vi "Close Group.vi"(8 "error in":errorcluster, 10 "Group":string, 11 "TDMS in":refnum<class "TDMS.lvclass">) -> (0 "error out":errorcluster, 3 "TDMS out":refnum<class "TDMS.lvclass">)   [LabVIEW 2019, in "TDMS.lvlib" / "TDMS.lvclass"]
uses:
  TDMS.lvclass
  TDMS.lvclass/TDMS.ctl
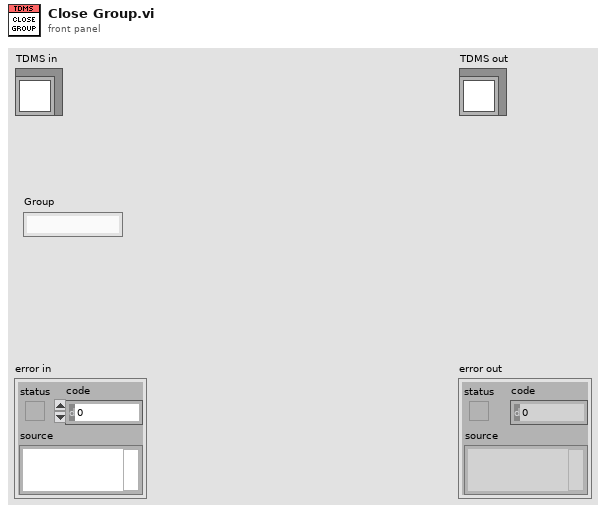
[diagram p1: front panel]
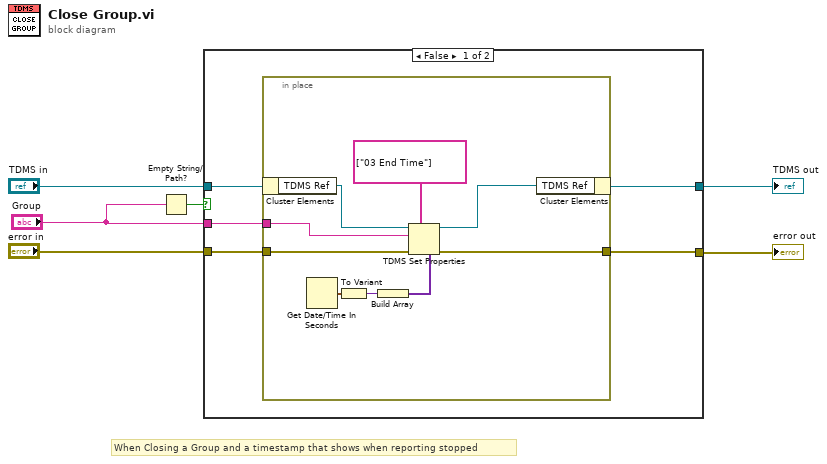
[diagram p0: block diagram]
diagram:
  # "When Closing a Group and a timestamp that shows when reporting stopped"
  n1 = Empty String/Path?(string/path="Group") -> (empty?=w2:bool)
  n2 = case shown="False" w2 {
    tunnel: [w11 w22] -> w6
    tunnel: "error in" -> [w10 w21]
    tunnel: [w9 w21] -> w4
    tunnel: "TDMS in" -> [w8 w22]
    tunnel: "Group" -> [w7 _]
    frame False {
      n3 = in-place {
        in-place-border: w10 -> [w16]
        in-place-border: [w18] -> w9
        in-place-border: w7 -> [w12]
        n4 = in-place-cluster #1(w8) -> ("TDMS Ref"=w20:refnum<k34>)
        n5 = Get Date/Time In Seconds() -> (seconds since 1Jan1904=w15:timestamp)
        n6 = To Variant(anything=w15) -> (Variant=w14:variant)
        n7 = Build Array(w14) -> (w17:variant[])
        n8 = TDMS Set Properties(5:w17, 7:string[] ["03 End Time"], 8:w16, 10:w12, 11:w20) -> (0:w18:errorcluster, 3:w19:refnum<k34>)  [unwired: 1 in, 2 out]
        n9 = in-place-cluster #1("TDMS Ref"=w19) -> (w11:refnum<class "TDMS.lvclass">)
      }
    }
    frame True {
    }
  }
  "error out" <- w4
  "TDMS out" <- w6
